vi "LJT4_avg_data.vi"(10 "data_raw":dbl[][](array[numeric])) -> (2 "data_avg":dbl[](array[numeric]))   [LabVIEW 2019]
uses:
  <vilib>/Analysis/baseanly.llb/Mean (DBL).vi
  <vilib>/Analysis/NI_AALBase.lvlib
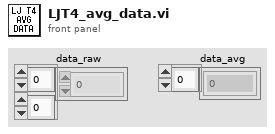
[diagram p1: front panel]
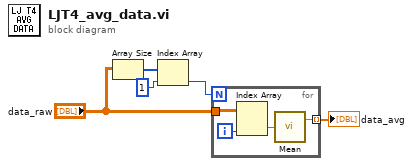
[diagram p0: block diagram]
diagram:
  n1 = Array Size(array="data_raw") -> (size(s)=w3:i32[])
  n2 = Index Array(array=w3, index=1) -> (element=w1:i32)
  n3 = for {
    N: w1 -> [_]
    tunnel: "data_raw" -> [w9]
    tunnel: [w6] -> w5 mode=indexing
    i -> [w8]
    n4 = Index Array(array=w9, index (col)=w8) -> (element=w7:dbl[])  [unwired: 1 in]
    n5 = call-poly <vilib>:"Mean.vi"("X"=w7) -> ("mean"=w6:dbl)  [unwired: 1 out]
  }
  "data_avg" <- w5
